vi "简易流程调试界面.vi"() -> ()   [LabVIEW 2016, in "斯坦道总磷.lvlib"]
uses:
  <vilib>/Utility/miscctls.llb/LVPointTypeDef.ctl
  <userlib>/_OpenG.lib/array/array.llb/Sort 1D Array (I32)__ogtk.vi
  <vilib>/Plasmionique/MB Master/MB_Master/MB_Master.lvclass
panel:
  in  "调试控件":enum32{"填充流程", "清洗流程", "测试流程", "排空流程", "其他流程"}(tab)
  in  "填充简易流程":i32(listbox)
  in  "清洗简易流程":i32(listbox)
  in  "测试简易流程":i32(listbox)
  in  "排空简易流程":i32(listbox)
  in  "其他简易流程":i32(listbox)
  in  "停止":bool
  in  "单步测试":bool
  out "注射器温度":sgl
  out "消解温度":sgl
  out "ADC":sgl
  out "F3":sgl format="%#.6f"
  out "F2":sgl format="%#.6f"
  out "F1":sgl format="%#.6f"
  out "F0":sgl format="%#.6f"
  in  "启动":bool
  in  "参数下拉列表":u16(ring) items=["总氮"=2]
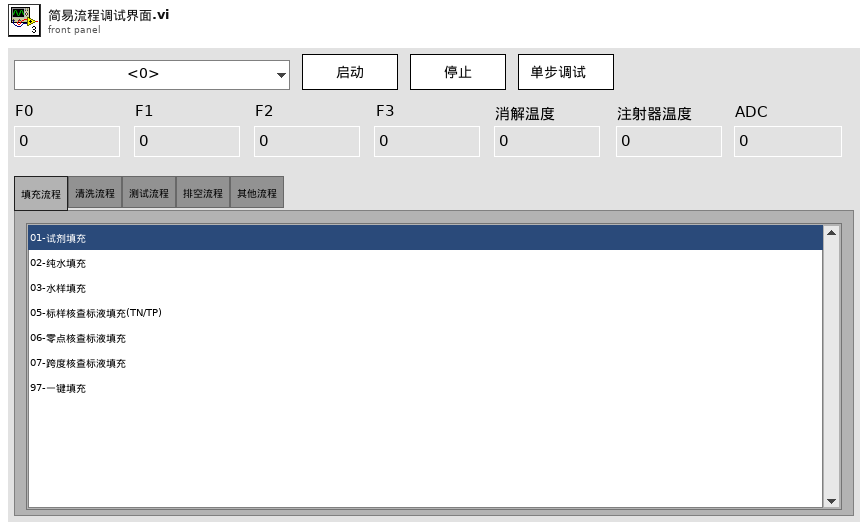
[diagram p1: front panel]
types:
  T1 = typedef "LVPointTypeDef.ctl" = cluster{"Horizontal":i16, "Vertical":i16}
  T2 = typedef "LVRectTypeDef.ctl" = cluster{"Left":i16, "Top":i16, "Right":i16, "Bottom":i16}
  T3 = typedef "LVStringsAndValuesArrayTypeDef_U16.ctl" = cluster{"String":string, "Value":u16}[]
  T4 = enum16{"跨度核查", "水样测量", "零点核查", "标样核查", "加标回收", "快捷测试", "空白校准", "标样校准"}
  T5 = cluster{"系统时间":timestamp, "工作状态":u16, "测量模式":enum16{"待机", "连续模式", "周期模式", "定点模式", "受控模式", "手动模式"}, "告警代码":u16, "故障代码":u16, "日志代码":u16, "软件版本":u16, "F0":sgl, "F1":sgl, "F2":sgl, "F3":sgl, "T":sgl, "H":sgl, "id":u16, "flowid":u16, "量程":u16, "总磷控温温度1":sgl, "营养盐控温温度2":sgl, "ADC":sgl}
  T6 = enum32{"Bad", "Idle", "Run top level", "Running"}
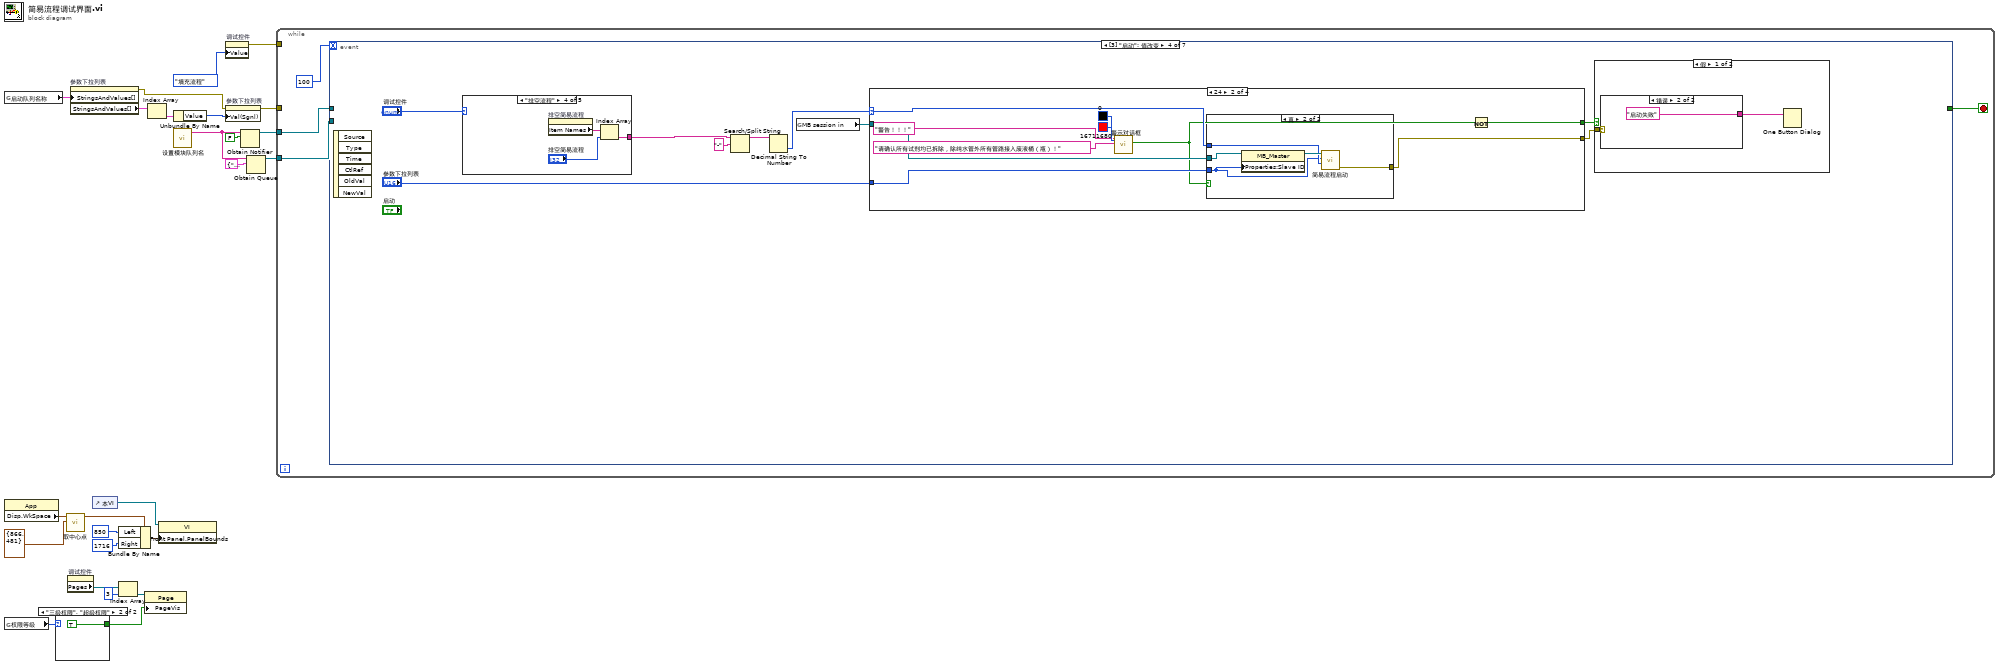
[diagram p0: block diagram]
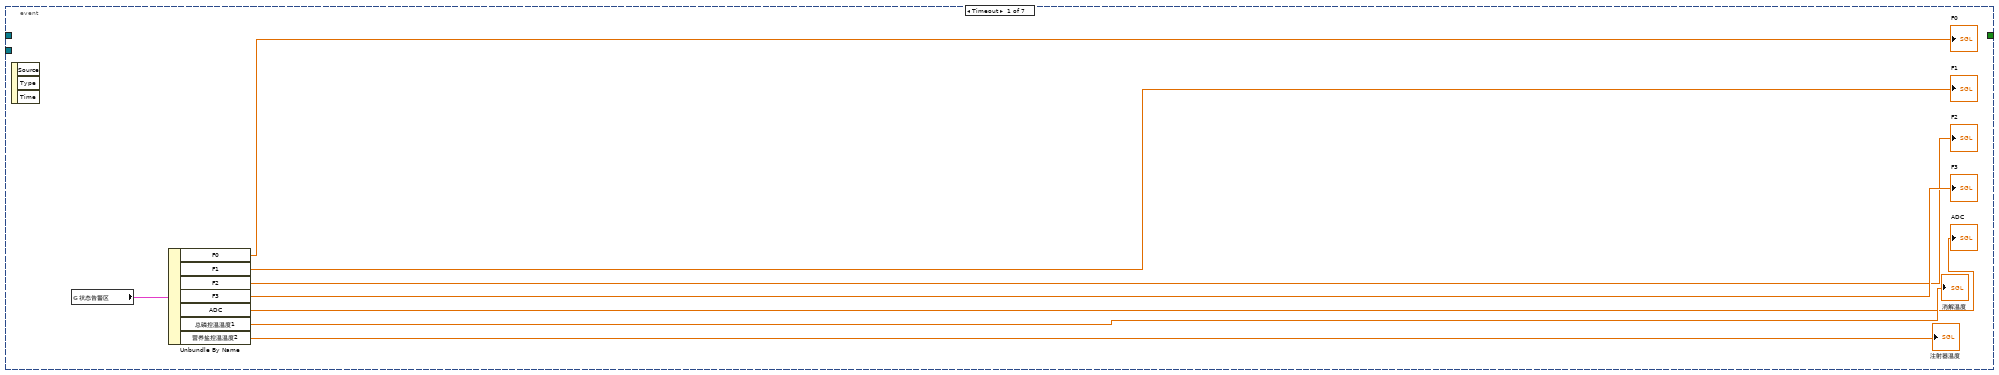
[diagram p3: hidden frame]
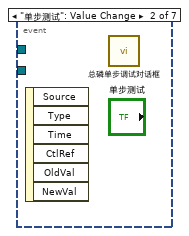
[diagram p4: hidden frame]
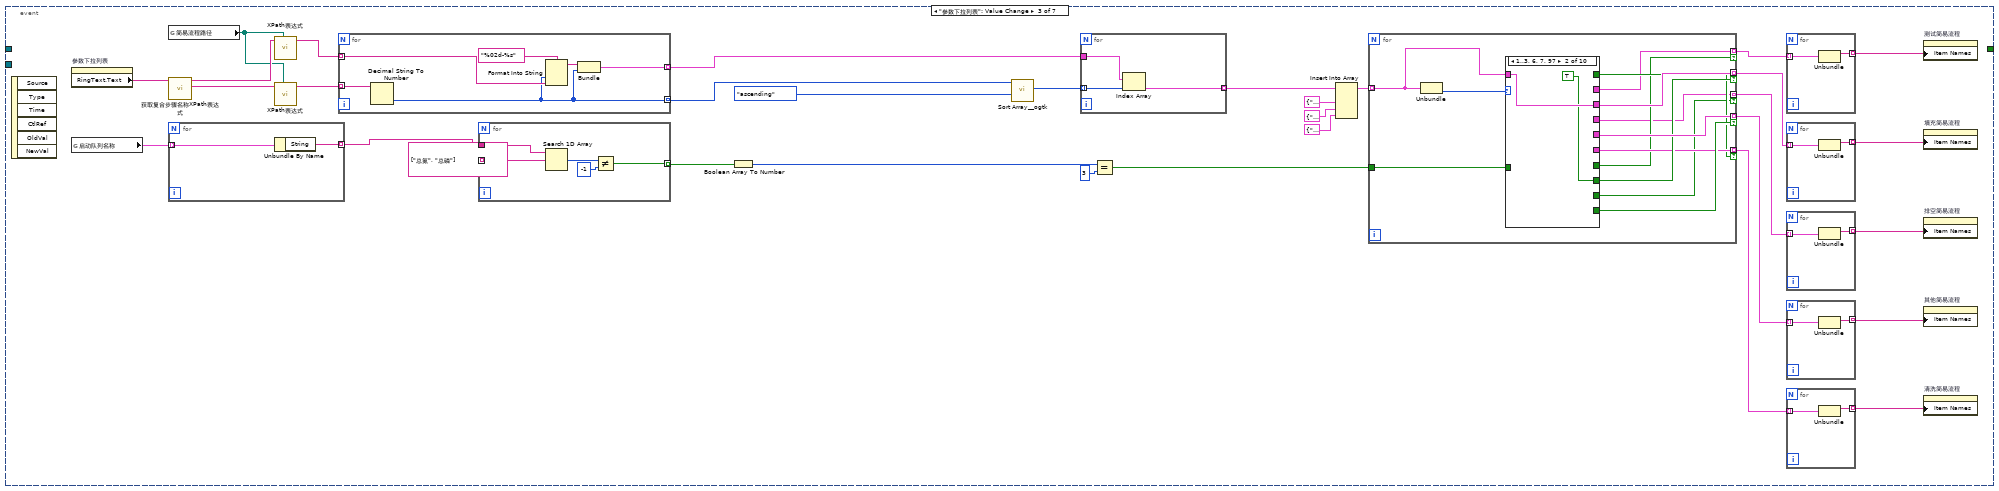
[diagram p5: hidden frame]
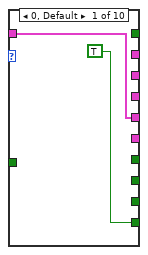
[diagram p6: hidden frame]
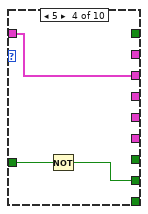
[diagram p8: hidden frame]
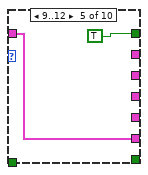
[diagram p9: hidden frame]
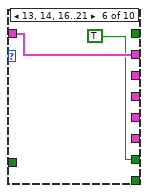
[diagram p10: hidden frame]
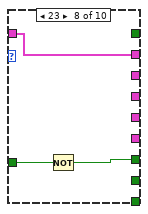
[diagram p12: hidden frame]
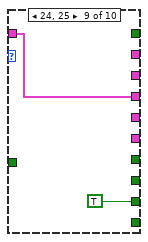
[diagram p13: hidden frame]
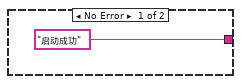
[diagram p15: hidden frame]
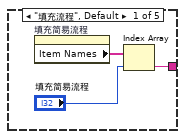
[diagram p17: hidden frame]
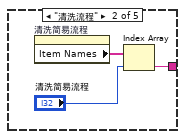
[diagram p18: hidden frame]
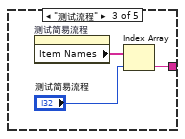
[diagram p19: hidden frame]
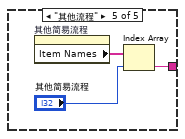
[diagram p20: hidden frame]
diagram:
  n1 = global read "总磷总氮断电保存全局变量.vi" "启动队列名称"() -> (w20:cluster{"String":string, "Value":u16}[])
  n2 = property class="App"() -> ("Disp.WkSpace"=w6:T2)  [unwired: 2 in, 2 out]
  n3 = global read "VAR总磷总氮全局变量.vi" "权限等级"() -> (w12:enum16{"一级权限", "二级权限", "三级权限", "超级权限"})
  n4 = case shown="\"三级权限\", \"超级权限\"" w12 {
    tunnel: [_ TRUE ("选项卡可见")] -> w8
    frame "一级权限", Default {
    }
    frame "三级权限", "超级权限" {
    }
  }
  n5 = call "取中心点.vi"("前面板窗口:最小尺寸"=T1 {"Horizontal"=866, "Vertical"=481}, "显示:主工作区"=w6) -> ("前面板窗口:窗口边界"=w4:T2)  [unwired: 9 in]
  n6 = property on="调试控件" class="TabCtl (严格)"() -> ("Pages"=w11:refnum<vi>[])  [unwired: 2 in, 2 out]
  n7 = property on="参数下拉列表" class="Ring (严格)"("StringsAndValues[]"=w20) -> (error out=w21:errorcluster, "StringsAndValues[]"=w24:T3)  [unwired: 2 in, 1 out]
  n8 = control-ref of="本VI"() -> (w7:refnum<vi>)
  n9 = Bundle By Name(cluster=w4, "Left"=i16 850, "Right"=i16 1716) -> (w3:T2)
  n10 = Index Array(array=w11, index=3 ("索引")) -> (element=w9:refnum<vi>)
  n11 = property class="Page"(reference=w9, "PageVis"=w8) -> ()  [unwired: 1 in, 2 out]
  n12 = Index Array(array=w24) -> (element=w23:cluster{"String":string, "Value":u16})  [unwired: 1 in]
  n13 = property class="VI"(reference=w7, "Front Panel.PanelBounds"=w3) -> ()  [unwired: 1 in, 2 out]
  n14 = Unbundle By Name(w23) -> ("Value"=w22:u16)
  n15 = call "设置模块队列名.vi"() -> ("Msg"=w17:string)  [unwired: 5 in]
  n16 = property on="调试控件" class="TabCtl (严格)"("Value"=enum32{"填充流程", "清洗流程", "测试流程", "排空流程", "其他流程"}."填充流程" ("调试控件")) -> (error out=w13:errorcluster)  [unwired: 2 in, 1 out]
  n17 = property on="参数下拉列表" class="Ring (严格)"(error in=w21, "Val(Sgnl)"=w22) -> (error out=w25:errorcluster)  [unwired: 1 in, 1 out]
  n18 = Obtain Notifier(name (unnamed)=w17, notification data type=FALSE) -> (notifier out=w16:refnum<notifier>)  [unwired: 2 in, 2 out]
  n19 = Obtain Queue(name (unnamed)=w17, element data type=cluster{"命令":string, "data":variant} {"命令"="", "data"=variant}) -> (queue out=w15:refnum<queue>)  [unwired: 3 in, 2 out]
  n20 = while {
    tunnel: w25 -> [_]
    tunnel: w16 -> [w28]
    tunnel: w15 -> [w27]
    tunnel: w13 -> [_]
    stop <- w30 stop-if-true
    n21 = event shown="[3] \"启动\": 值改变" {
      selector: _ -> [_ _ _ _ _ _ _]
      dyn-events: _ -> [_ _ _ _ _ _ _]
      timeout: 100 -> [_ _ _ _ _ _ _]
      tunnel: [_ _ _ _ _ _ TRUE] -> w30
      tunnel: w28 -> [_ _ _ _ _ w201 _]
      tunnel: w27 -> [_ _ _ _ _ w200 _]
      event Timeout {
        n22 = event-data() -> ()  [unwired: 1 in, 3 out]
        n23 = global read "VAR总磷总氮全局变量.vi" "状态告警区"() -> (w38:T5)
        n24 = Unbundle By Name(w38) -> ("F0"=→"F0":sgl, "F1"=→"F1":sgl, "F2"=→"F2":sgl, "F3"=→"F3":sgl, "ADC"=→"ADC":sgl, "总磷控温温度1"=→"消解温度":sgl, "营养盐控温温度2"=→"注射器温度":sgl)
      }
      event "单步测试": Value Change {
        n25 = event-data() -> ()  [unwired: 1 in, 6 out]
        n26 = call "总磷单步调试对话框.vi"() -> ()  [unwired: 12 in]
      }
      event "参数下拉列表": Value Change {
        n27 = event-data() -> ()  [unwired: 1 in, 6 out]
        n28 = property on="参数下拉列表" class="Ring (严格)"() -> ("RingText.Text"=w70:string)  [unwired: 2 in, 2 out]
        n29 = global read "总磷总氮断电保存全局变量.vi" "启动队列名称"() -> (w45:cluster{"String":string, "Value":u16}[])
        n30 = global read "总磷总氮断电保存全局变量.vi" "简易流程路径"() -> (w65:path)
        n31 = call "获取复合步骤名称XPath表达式.vi"("查询参数"=w70) -> ("FlowId"=w68:string, "name"=w69:string)  [unwired: 9 in]
        n32 = for {
          tunnel: w45 -> [w72] mode=indexing
          tunnel: [w71] -> w44 mode=indexing
          n33 = Unbundle By Name(w72) -> ("String"=w71:string)
        }
        n34 = call "XPath表达式.vi"("添加的路径"=w65, "XPath expression"=w69) -> ("数组"=w67:string[])  [unwired: 9 in]
        n35 = call "XPath表达式.vi"("添加的路径"=w65, "XPath expression"=w68) -> ("数组"=w66:string[])  [unwired: 9 in]
        n36 = for {
          tunnel: w67 -> [w127] mode=indexing
          tunnel: w66 -> [w130] mode=indexing
          tunnel: [w129] -> w62 mode=indexing
          tunnel: [w125] -> w64 mode=indexing
          n37 = Decimal String To Number(string=w130) -> (number=w125:i32)  [unwired: 2 in, 1 out]
          n38 = Format Into String(format string="%02d-%s" ("格式字符串"), w125, w127) -> (resulting string=w126:string)  [unwired: 2 in, 1 out]
          n39 = Bundle(w126, w125) -> (w129:cluster{string, i32})  [unwired: 1 in]
        }
        n40 = for {
          tunnel: string[] ["总氮", "总磷"] -> [w76] mode=indexing
          tunnel: w44 -> [w77]
          tunnel: [w73] -> w43 mode=indexing
          n41 = Search 1D Array(1D array=w77, element=w76) -> (index of element=w75:i32)  [unwired: 1 in]
          n42 = Not Equal?(x=w75, y=-1) -> (x != y?=w73:bool)
        }
        n43 = Boolean Array To Number(Boolean array=w43) -> (number=w42:u32)
        n44 = call-poly <userlib>:"Sort Array__ogtk.vi"("Order"=enum16{"ascending", "descending"}."ascending", "Array in"=w64) -> ("Sorted Pointers"=w61:i32[])  [unwired: 8 in, 1 out]
        n45 = for {
          tunnel: w62 -> [w124]
          tunnel: w61 -> [w123] mode=indexing
          tunnel: [w122] -> w56 mode=indexing
          n46 = Index Array(array=w124, index=w123) -> (element=w122:cluster{string, i32})
        }
        n47 = Equal?(x=w42, y=u32 3) -> (x = y?=w40:bool)
        n48 = Insert Into Array(array=w56, new element #1=cluster{string, i32} {"97-一键填充", 97} ("新元素/子数组"), new element #2=cluster{string, i32} {"98-快捷测试（低量程）", 98} ("新元素/子数组"), new element #3=cluster{string, i32} {"99-快捷测试（高量程）", 99} ("新元素/子数组")) -> (w55:cluster{string, i32}[])  [unwired: 1 in]
        n49 = for {
          tunnel: w55 -> [w99] mode=indexing
          tunnel: [w98] -> w48 mode=indexing if=w97
          tunnel: [w96] -> w58 mode=indexing if=w95
          tunnel: [w94] -> w54 mode=indexing if=w93
          tunnel: [w92] -> w52 mode=indexing if=w91
          tunnel: [w90] -> w50 mode=indexing if=w89
          tunnel: w40 -> [w88]
          n50 = Unbundle(w99) -> (w100:i32)  [unwired: 1 out]
          n51 = case shown="1..3, 6, 7, 97" w100 {
            tunnel: [w102 _ _ _ _ _ _ _ _ _] -> w98
            tunnel: w99 -> [w102 w104 w106 w109 w111 w113 w115 w118 w120 w121]
            tunnel: [TRUE _ _ _ _ _ _ _ _ _] -> w97
            tunnel: [_ w104 w106 w109 _ _ _ _ _ _] -> w96
            tunnel: [_ TRUE w105 w107 _ _ _ _ _ _] -> w95
            tunnel: [_ _ _ _ w111 _ _ _ _ _] -> w94
            tunnel: [_ _ _ _ TRUE _ _ _ _ _] -> w93
            tunnel: [_ _ _ _ _ w113 w115 w118 _ _] -> w92
            tunnel: [_ _ _ _ _ TRUE w114 w116 _ _] -> w91
            tunnel: [_ _ _ _ _ _ _ _ w120 w121] -> w90
            tunnel: [_ _ _ _ _ _ _ _ TRUE _] -> w89
            tunnel: w88 -> [_ _ w105 w108 _ _ w114 w117 _ _]
            frame 0, Default {
            }
            frame 1..3, 6, 7, 97 {
            }
            frame 4 {
            }
            frame 5 {
              n52 = Not(x=w108) -> (.not. x?=w107:bool)
            }
            frame 9..12 {
            }
            frame 13, 14, 16..21 {
            }
            frame 22 {
            }
            frame 23 {
              n53 = Not(x=w117) -> (.not. x?=w116:bool)
            }
            frame 24, 25 {
            }
            frame 8, 15 {
            }
          }
        }
        n54 = for {
          tunnel: w52 -> [w83] mode=indexing
          tunnel: [w82] -> w51 mode=indexing
          n55 = Unbundle(w83) -> (w82:string)  [unwired: 1 out]
        }
        n56 = for {
          tunnel: w58 -> [w87] mode=indexing
          tunnel: [w86] -> w57 mode=indexing
          n57 = Unbundle(w87) -> (w86:string)  [unwired: 1 out]
        }
        n58 = for {
          tunnel: w50 -> [w81] mode=indexing
          tunnel: [w80] -> w49 mode=indexing
          n59 = Unbundle(w81) -> (w80:string)  [unwired: 1 out]
        }
        n60 = for {
          tunnel: w48 -> [w79] mode=indexing
          tunnel: [w78] -> w47 mode=indexing
          n61 = Unbundle(w79) -> (w78:string)  [unwired: 1 out]
        }
        n62 = for {
          tunnel: w54 -> [w85] mode=indexing
          tunnel: [w84] -> w53 mode=indexing
          n63 = Unbundle(w85) -> (w84:string)  [unwired: 1 out]
        }
        n64 = property on="测试简易流程" class="LstBox (严格)"("Item Names"=w51) -> ()  [unwired: 2 in, 2 out]
        n65 = property on="填充简易流程" class="LstBox (严格)"("Item Names"=w57) -> ()  [unwired: 2 in, 2 out]
        n66 = property on="排空简易流程" class="LstBox (严格)"("Item Names"=w49) -> ()  [unwired: 2 in, 2 out]
        n67 = property on="其他简易流程" class="LstBox (严格)"("Item Names"=w47) -> ()  [unwired: 2 in, 2 out]
        n68 = property on="清洗简易流程" class="LstBox (严格)"("Item Names"=w53) -> ()  [unwired: 2 in, 2 out]
      }
      event "启动": Value Change {
        n69 = event-data() -> ()  [unwired: 1 in, 6 out]
        n70 = case shown="\"排空流程\"" "调试控件" {
          tunnel: [w144 w147 w150 w153 w156] -> w135
          frame "填充流程", Default {
            n71 = property on="填充简易流程" class="LstBox (严格)"() -> ("Item Names"=w146:string[])  [unwired: 2 in, 2 out]
            n72 = Index Array(array=w146, index="填充简易流程") -> (element=w144:string)
          }
          frame "清洗流程" {
            n73 = property on="清洗简易流程" class="LstBox (严格)"() -> ("Item Names"=w149:string[])  [unwired: 2 in, 2 out]
            n74 = Index Array(array=w149, index="清洗简易流程") -> (element=w147:string)
          }
          frame "测试流程" {
            n75 = property on="测试简易流程" class="LstBox (严格)"() -> ("Item Names"=w152:string[])  [unwired: 2 in, 2 out]
            n76 = Index Array(array=w152, index="测试简易流程") -> (element=w150:string)
          }
          frame "排空流程" {
            n77 = property on="排空简易流程" class="LstBox (严格)"() -> ("Item Names"=w155:string[])  [unwired: 2 in, 2 out]
            n78 = Index Array(array=w155, index="排空简易流程") -> (element=w153:string)
          }
          frame "其他流程" {
            n79 = property on="其他简易流程" class="LstBox (严格)"() -> ("Item Names"=w158:string[])  [unwired: 2 in, 2 out]
            n80 = Index Array(array=w158, index="其他简易流程") -> (element=w156:string)
          }
        }
        n81 = Search/Split String(string=w135, search string/char (-)="-" ("搜索字符串/字符(-)")) -> (substring before match=w133:string)  [unwired: 1 in, 2 out]
        n82 = Decimal String To Number(string=w133) -> (number=w132:i32)  [unwired: 2 in, 1 out]
        n83 = global read "VAR总磷总氮全局变量.vi" "MB session in"() -> (w138:refnum<class "MB_Master.lvclass">)
        n84 = case shown="24" w132 {
          selector: w132 -> [w161 w172 _ w193]
          tunnel: [w163 w173 _ w197] -> w139
          tunnel: w138 -> [w160 w171 _ w196]
          tunnel: "参数下拉列表" -> [w159 w170 w179 w195]
          tunnel: [_ w169 _ _] -> w131
          frame 0, Default {
            n85 = property class="MB_Master"(reference=w160, "Properties:Slave ID"=w159) -> (reference out=w162:refnum<class "MB_Master.lvclass">)  [unwired: 1 in, 1 out]
            n86 = call "简易流程启动.vi"("简易流程"=w161, "参数Id"=w159, "MB session in"=w162) -> ("error out"=w163:errorcluster)  [unwired: 7 in, 1 out]
          }
          frame 24 {
            n87 = call "警示对话框.vi"("副标题颜色"=u32 0, "主标题颜色"=u32 16711680, "副标题"="请确认所有试剂均已拆除，除纯水管外所有管路接入废液桶（瓶）！" ("消息"), "主标题"="警告！！！" ("消息")) -> ("check"=w164:bool)  [unwired: 7 in]
            n88 = case shown="真" w164 {
              tunnel: [_ w178] -> w173
              tunnel: w172 -> [_ w176]
              tunnel: w171 -> [_ w175]
              tunnel: w170 -> [_ w174]
              frame False {
              }
              frame True {
                n89 = property class="MB_Master"(reference=w175, "Properties:Slave ID"=w174) -> (reference out=w177:refnum<class "MB_Master.lvclass">)  [unwired: 1 in, 1 out]
                n90 = call "简易流程启动.vi"("简易流程"=w176, "参数Id"=w174, "MB session in"=w177) -> ("error out"=w178:errorcluster)  [unwired: 7 in, 1 out]
              }
            }
            n91 = Not(x=w164) -> (.not. x?=w169:bool)
          }
          frame 97 {
            n92 = vi-ref "一键清洗流程.vi"() -> (w180:refnum<vi>)
            n93 = property class="VI"(reference=w180) -> ("Name"=w181:string, "Exec.State"=w182:T6)  [unwired: 1 in, 2 out]
            n94 = case shown="\"Idle\"" w182 {
              tunnel: w181 -> [_ w191]
              tunnel: w179 -> [_ w184]
              frame "Bad", Default {
              }
              frame "Idle" {
                n95 = Open VI Reference(type specifier VI Refnum (for type only)=refnum<vi> refnum, vi path=w191, options=128 ("选项")) -> (vi reference=w188:refnum<vi>, error out=w186:errorcluster)  [unwired: 3 in]
                n96 = property on="填充简易流程" class="LstBox (严格)"() -> ("Item Names"=w183:string[])  [unwired: 2 in, 2 out]
                n97 = call-by-ref "开始异步调用"(reference=w188, error in=w186, "项名"=w183, "参数下拉列表"=w184) -> (reference out=w187:refnum<vi>, error out=w185:errorcluster)  [unwired: 10 in]
                n98 = Close Reference(reference=w187, error in (no error)=w185) -> ()  [unwired: 1 out]
              }
            }
          }
          frame 98, 99 {
            n99 = case shown="98, 默认" w193 {
              tunnel: [enum16{"低量程", "高量程"}."低量程" ("量程下拉列表") enum16{"低量程", "高量程"}."高量程" ("量程下拉列表")] -> w192
              frame 98, Default {
              }
              frame 99 {
              }
            }
            n100 = call "非国标启动命令.vi"("参数下拉列表"=w195, "量程下拉列表"=w192, "测量模式"=T4."快捷测试", "MB session in"=w196) -> ("error out"=w197:errorcluster)  [unwired: 6 in, 1 out]
          }
        }
        n101 = case shown="假" w131 {
          tunnel: w139 -> [w141 _]
          frame False {
            n102 = case shown="错误" w141 {
              tunnel: ["启动成功" "启动失败"] -> w140
              frame No Error {
              }
              frame Error {
              }
            }
            n103 = One Button Dialog(message=w140) -> ()  [unwired: 1 in, 1 out]
          }
          frame True {
          }
        }
      }
      event "排空简易流程": Mouse Down {
        n104 = event-data() -> ()  [unwired: 1 in, 6 out]
      }
      event "停止": Value Change {
        n105 = event-data() -> ()  [unwired: 1 in, 6 out]
        n106 = Send Notification(notification=TRUE ("通知"), notifier=w201) -> ()  [unwired: 1 in, 2 out]
        n107 = Enqueue Element(queue=w200, element=cluster{"命令":string, "data":variant} {"命令"="启动", "data"=variant(cluster{"站号":u16, "控制命令输出":u16[]} {"站号"=1, "控制命令输出"=[2816]})} ("元素")) -> (queue out=w203:refnum<queue>)  [unwired: 2 in, 2 out]
        n108 = Enqueue Element(queue=w203, element=cluster{"命令":string, "data":variant} {"命令"="启动", "data"=variant(cluster{"站号":u16, "控制命令输出":u16[]} {"站号"=2, "控制命令输出"=[2816]})} ("元素")) -> ()  [unwired: 2 in, 3 out]
      }
      event Panel Close {
        n109 = event-data() -> ()  [unwired: 1 in, 3 out]
      }
    }
  }
